vi "wave-to-pixelSD.vi"(1 "Wave":dbl format="%#_13g") -> (0 "Wave, pixel":dbl)   [LabVIEW 2015]
uses:
  globalVarSD.vi
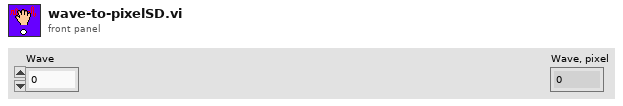
[diagram p1: front panel]
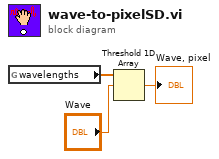
[diagram p0: block diagram]
diagram:
  n1 = global read "globalVarSD.vi" "wavelengths"() -> (w1:dbl[])
  n2 = Threshold 1D Array(2:"Wave", 3:w1) -> (0:→"Wave, pixel":dbl)  [unwired: 1 in]
